vi "Voltage Output Test.vi"(7 "Test Socket (0)":i32, 8 "DMM Channel":i32=2, 9 "Line In":dbl, 10 "Power Supply In":string, 11 "DMM In":string) -> (0 "error out":errorcluster, 3 "Output Voltage":dbl)   [LabVIEW 2013]
doc: "Measures the output RMS voltage when providing an input voltage from a specified pin."
uses:
  Shipped/Exercises/Driver Simulation API/Support/DMM/Signal Types.ctl
  Shipped/Exercises/Driver Simulation API/Support/Power Supply.lvlib
  Shipped/Exercises/Driver Simulation API/Support/DMM.lvlib
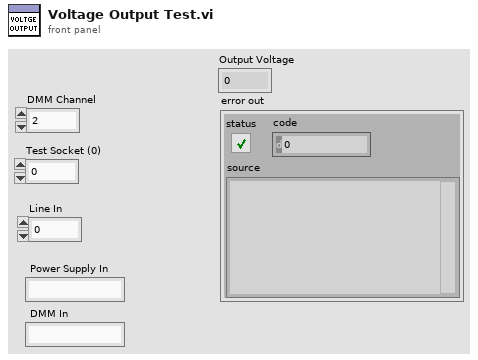
[diagram p1: front panel]
types:
  T1 = typedef "Driver Simulation.lvlib/DMM.lvlib/Signal Types.ctl" = enum16{"DC", "AC"}
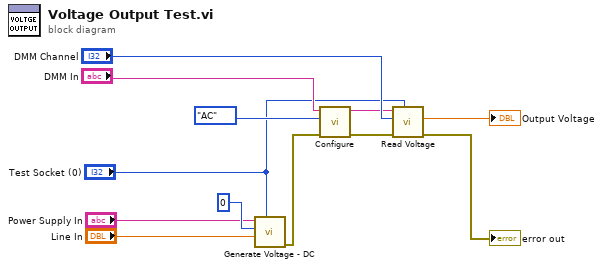
[diagram p0: block diagram]
diagram:
  n1 = call "Generate Voltage - DC.vi"("Test Socket (0)"="Test Socket (0)", "outputVoltage"="Line In", "channel"=0 ("Power Supply Channel"), "Power Supply in"="Power Supply In") -> ("error out"=w6:errorcluster)  [unwired: 6 in, 1 out]
  n2 = call "Configure.vi"("error in (no error)"=w6, "signalType"=Signal_Types."AC", "DMM in"="DMM In") -> ("error out"=w5:errorcluster, "DMM out"=w2:string)  [unwired: 7 in]
  n3 = call "Read Voltage.vi"("Test Socket (0)"="Test Socket (0)", "error in (no error)"=w5, "Channel"="DMM Channel", "DMM in"=w2) -> ("error out"=→"error out":errorcluster, "Voltage"=→"Output Voltage":dbl)  [unwired: 5 in, 1 out]
